vi "NewCreatorA.vi"(8 "error in (no error)":errorcluster) -> (0 "error out":errorcluster, 3 "CreatorA":refnum<class "CreatorA.lvclass">)   [LabVIEW 2020, in "FactoryMethod.lvlib" / "FactoryMethodLazyEvaluation.lvlib" / "CreatorA.lvclass"]
uses:
  CreatorA.lvclass
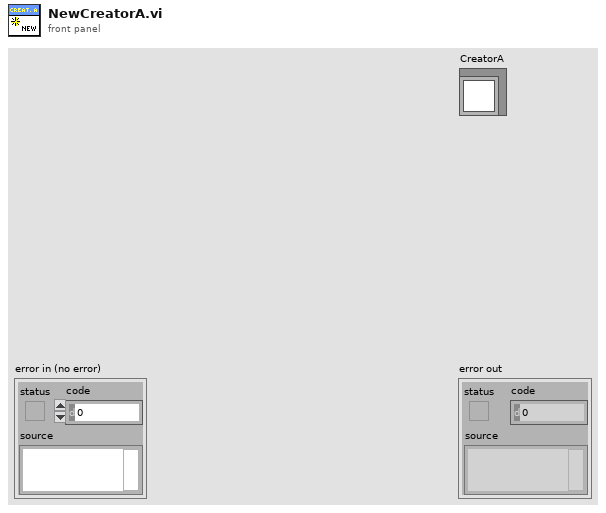
[diagram p1: front panel]
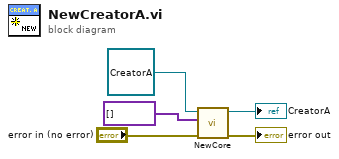
[diagram p0: block diagram]
diagram:
  n1 = call-dynamic "NewCore.vi"("error in (no error)"="error in (no error)", "ParamsArray"=variant[] [], "CreatorA"=refnum<class "CreatorA.lvclass"> refnum ("ConcreteCreatorA in")) -> ("error out"=→"error out":errorcluster, "CreatorA"=→"CreatorA":refnum<class "CreatorA.lvclass">)  [unwired: 7 in]
